vi "_Initialize Sequence.vi"(8 "error in (no error)":errorcluster, 11 "Sequencer in":refnum<class "Sequencer.lvclass">) -> (0 "error out":errorcluster, 3 "Sequencer out":refnum<class "Sequencer.lvclass">)   [LabVIEW 2015, in "Sequencer.lvlib" / "Sequencer.lvclass"]
uses:
  Sequencer.lvclass
  Sequencer.lvclass/Sequencer.ctl
  Read AO DAQChannels.vi
  Read AO Waveforms.vi
  Read AOChConfigs.vi
  SequencerConfig.lvclass
  Analog Output Channel/AOChConfig.lvclass
  SequencerInfo.lvclass
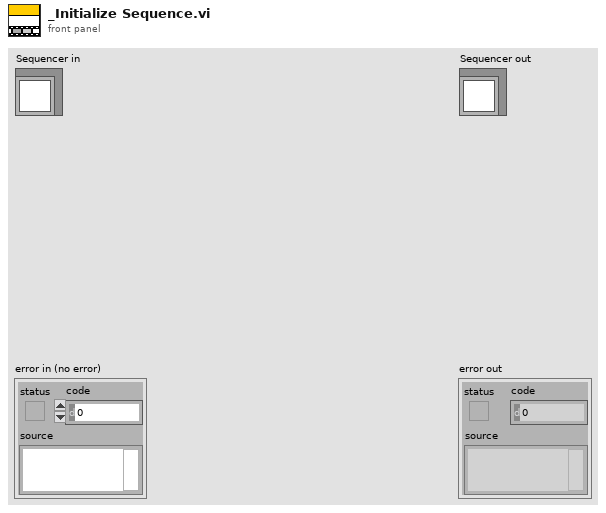
[diagram p1: front panel]
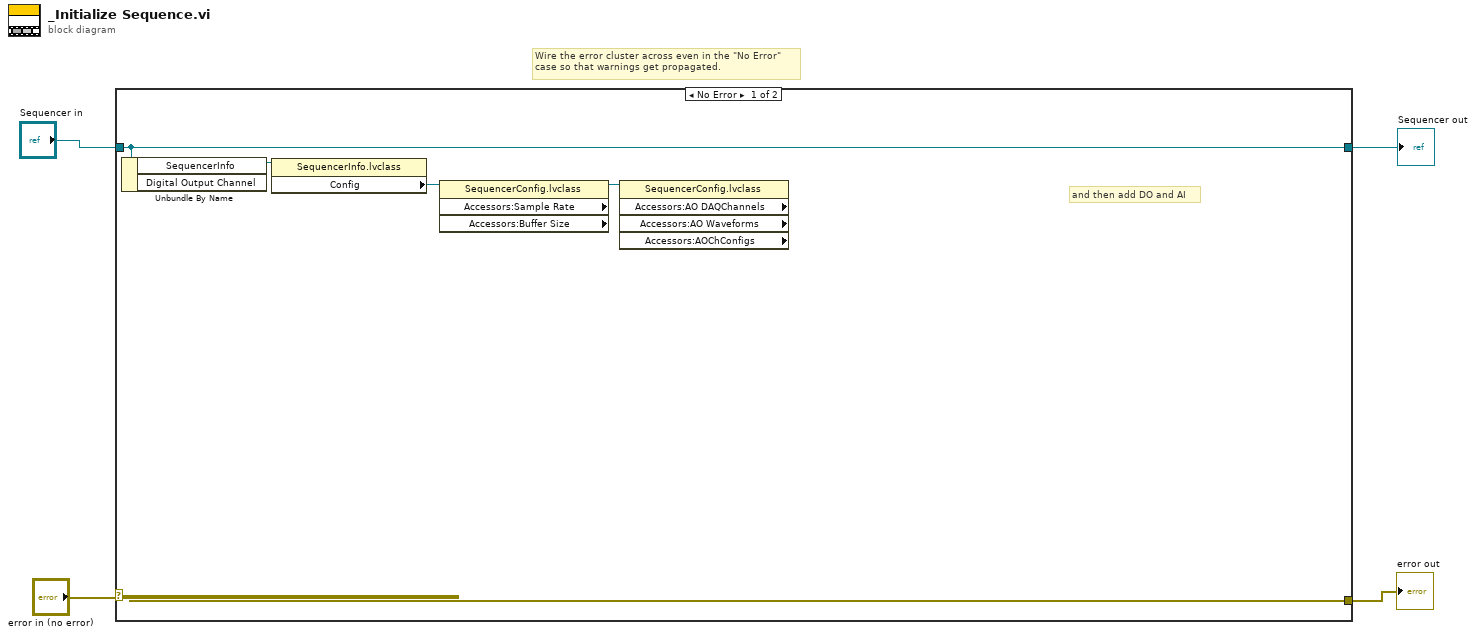
[diagram p0: block diagram]
diagram:
  # "Wire the error cluster across even in the \"No Error\"\ncase so that warnings get propagated."
  n1 = case shown="No Error" "error in (no error)" {
    selector: "error in (no error)" -> [w5 w11]
    tunnel: [w5 w11] -> w3
    tunnel: [w9 w10] -> w1
    tunnel: "Sequencer in" -> [w9 w10]
    frame No Error {
      # "and then add DO and AI"
      n2 = Unbundle By Name(w9) -> ("SequencerInfo"=w8:refnum<class "SequencerInfo.lvclass">)  [unwired: 1 out]
      n3 = property class="SequencerInfo.lvclass"(reference=w8) -> ("Config"=w7:refnum<class "SequencerConfig.lvclass">)  [unwired: 1 in, 2 out]
      n4 = property class="SequencerConfig.lvclass" props=["Accessors:Sample Rate", "Accessors:Buffer Size"](reference=w7) -> (reference out=w6:refnum<class "SequencerConfig.lvclass">)  [unwired: 1 in, 3 out]
      n5 = property class="SequencerConfig.lvclass" props=["Accessors:AO DAQChannels", "Accessors:AO Waveforms", "Accessors:AOChConfigs"](reference=w6) -> ()  [unwired: 1 in, 5 out]
    }
    frame Error {
    }
  }
  "error out" <- w3
  "Sequencer out" <- w1
